vi "Set motor Duty cycle.vi"(8 "error in (no error)":errorcluster, 9 "Tipo de control":T2, 10 "Parametros de control":T1={"Setpoint"=0.0, "PV"=0.0, "Frecuencia PWM"=0.0, "Ciclo de trabajo PWM"=2.5e-06, "V. histeresis (grados)"=0.0, "Ganacias PID"={"proportional gain (Kc)"=1.0, "integral time (Ti, min)"=0.01, "derivative time (Td, min)"=0.0}, "Ref array"=[]} {"Ciclo de trabajo PWM" min=2.5e-06 max=1.0 step=0.1}) -> (0 "error out":errorcluster, 3 "Salida a motores":cluster{"duty cycle":dbl, "frequency":dbl}[](array[cluster]))   [LabVIEW 2018]
uses:
  <vilib>/addons/control/pid/NI_PID_pid.lvlib
  <vilib>/addons/control/pid/pid.llb/PID Percentage to EGU (DBL).vi
  <vilib>/addons/control/pid/_prctrl compat.llb/PID (Compatibility).vi
  <vilib>/addons/control/pid/NI_PID__prctrl compat.lvlib
  typedef/Selector control.ctl
  typedef/Parametros control.ctl
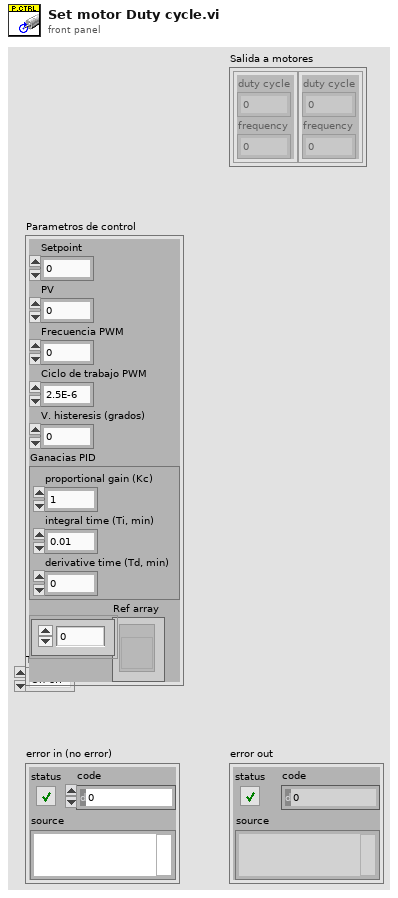
[diagram p1: front panel]
types:
  T1 = typedef "Parametros control.ctl" = cluster{"Setpoint":dbl, "PV":dbl, "Frecuencia PWM":dbl, "Ciclo de trabajo PWM":dbl, "V. histeresis (grados)":dbl, "Ganacias PID":cluster{"proportional gain (Kc)":dbl, "integral time (Ti, min)":dbl, "derivative time (Td, min)":dbl}, "Ref array":refnum<vi>[]}
  T2 = typedef "Selector control.ctl" = enum16{"On-off", "On-off hist.", "PID"}
  T3 = cluster{"sp low":dbl, "sp high":dbl, "out low":dbl, "out high":dbl, "hold (F)":bool, "auto (T)":bool, "pro. band (F)":bool, "reverse acting (T)":bool, "beta":dbl, "linearity":dbl, "dt (s)":dbl}
  T4 = cluster{"proportional gain (Kc)":dbl, "integral time (Ti, min)":dbl, "derivative time (Td, min)":dbl}
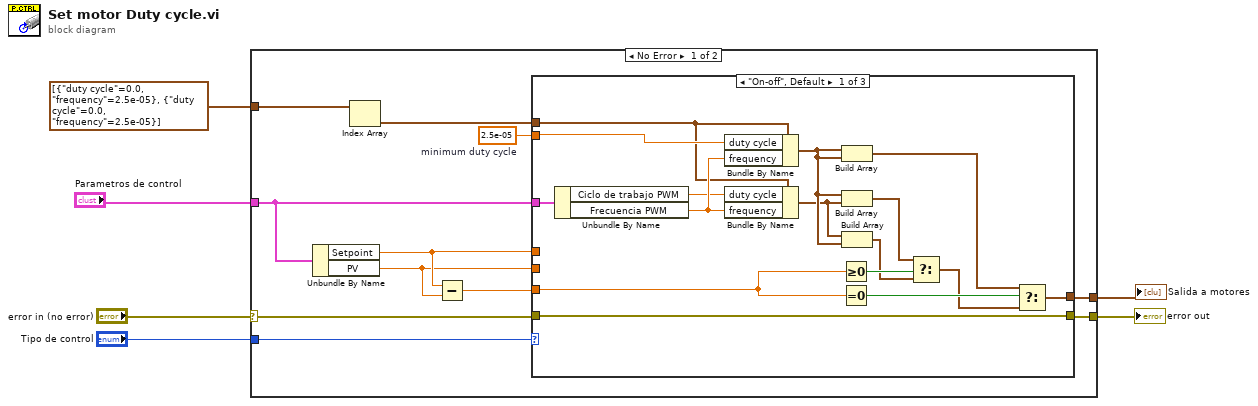
[diagram p0: block diagram]
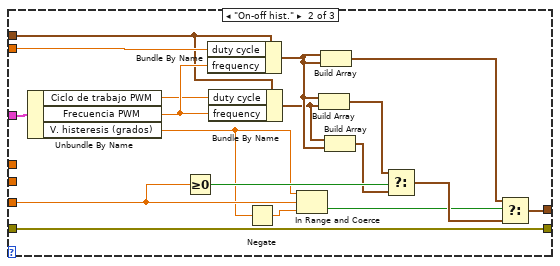
[diagram p2: hidden frame]
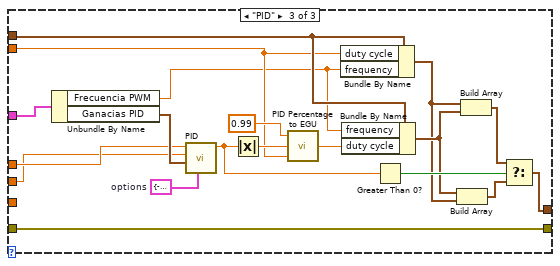
[diagram p3: hidden frame]
diagram:
  n1 = case shown="No Error" "error in (no error)" {
    selector: "error in (no error)" -> [w16 w72]
    tunnel: [w15 w72] -> w5
    tunnel: cluster{"duty cycle":dbl, "frequency":dbl}[] [{"duty cycle"=0.0, "frequency"=2.5e-05}, {"duty cycle"=0.0, "frequency"=2.5e-05}] ("data") -> [w10 w71]
    tunnel: [w17 w71] -> w3
    tunnel: "Parametros de control" -> [w13 _]
    tunnel: "Tipo de control" -> [w14 _]
    frame No Error {
      w11 = 2.5e-05  # minimum duty cycle
      n2 = Unbundle By Name(w13) -> ("Setpoint"=w9:dbl, "PV"=w8:dbl)
      n3 = Index Array(array=w10) -> (element=w7:cluster{"duty cycle":dbl, "frequency":dbl})  [unwired: 1 in]
      n4 = Subtract(x=w9, y=w8) -> (x-y=w12:dbl)
      n5 = case shown="\"On-off\", Default" w14 {
        tunnel: w12 -> [w31 w38 _]
        tunnel: [w22 w42 w63] -> w17
        tunnel: w13 -> [w21 w41 w70]
        tunnel: w16 -> [w20 w40 w68]
        tunnel: [w20 w40 w68] -> w15
        tunnel: w11 -> [w19 w35 w58]
        tunnel: w9 -> [_ _ w60]
        tunnel: w8 -> [_ _ w59]
        tunnel: w7 -> [w18 w34 w66]
        frame "On-off", Default {
          n6 = Unbundle By Name(w21) -> ("Ciclo de trabajo PWM"=w29:dbl, "Frecuencia PWM"=w30:dbl)
          n7 = Bundle By Name(cluster=w18, "duty cycle"=w19, "frequency"=w30) -> (w26:cluster{"duty cycle":dbl, "frequency":dbl})
          n8 = Bundle By Name(cluster=w18, "duty cycle"=w29, "frequency"=w30) -> (w25:cluster{"duty cycle":dbl, "frequency":dbl})
          n9 = Greater Or Equal To 0?(x=w31) -> (x >= 0?=w32:bool)
          n10 = Equal To 0?(x=w31) -> (x = 0?=w33:bool)
          n11 = Build Array(w26, w26) -> (w28:cluster{"duty cycle":dbl, "frequency":dbl}[])
          n12 = Build Array(w26, w25) -> (w27:cluster{"duty cycle":dbl, "frequency":dbl}[])
          n13 = Build Array(w25, w26) -> (w24:cluster{"duty cycle":dbl, "frequency":dbl}[])
          n14 = Select(t=w27, s=w32, f=w24) -> (s? t:f=w23:cluster{"duty cycle":dbl, "frequency":dbl}[])
          n15 = Select(t=w28, s=w33, f=w23) -> (s? t:f=w22:cluster{"duty cycle":dbl, "frequency":dbl}[])
        }
        frame "On-off hist." {
          n16 = Unbundle By Name(w41) -> ("Ciclo de trabajo PWM"=w49:dbl, "Frecuencia PWM"=w50:dbl, "V. histeresis (grados)"=w36:dbl)
          n17 = Greater Or Equal To 0?(x=w38) -> (x >= 0?=w51:bool)
          n18 = Bundle By Name(cluster=w34, "duty cycle"=w35, "frequency"=w50) -> (w46:cluster{"duty cycle":dbl, "frequency":dbl})
          n19 = Bundle By Name(cluster=w34, "duty cycle"=w49, "frequency"=w50) -> (w45:cluster{"duty cycle":dbl, "frequency":dbl})
          n20 = Negate(x=w36) -> (-x=w37:dbl)
          n21 = In Range and Coerce(upper limit=w36, x=w38, lower limit=w37) -> (In Range?=w39:bool)  [unwired: 1 out]
          n22 = Build Array(w46, w45) -> (w47:cluster{"duty cycle":dbl, "frequency":dbl}[])
          n23 = Build Array(w46, w46) -> (w48:cluster{"duty cycle":dbl, "frequency":dbl}[])
          n24 = Build Array(w45, w46) -> (w44:cluster{"duty cycle":dbl, "frequency":dbl}[])
          n25 = Select(t=w47, s=w51, f=w44) -> (s? t:f=w43:cluster{"duty cycle":dbl, "frequency":dbl}[])
          n26 = Select(t=w48, s=w39, f=w43) -> (s? t:f=w42:cluster{"duty cycle":dbl, "frequency":dbl}[])
        }
        frame "PID" {
          w54 = T3 {"sp low"=-180.0, "sp high"=180.0, "out low"=-170.0, "out high"=170.0, "hold (F)"=FALSE, "auto (T)"=TRUE, "pro. band (F)"=FALSE, "reverse acting (T)"=TRUE, "beta"=1.0, "linearity"=1.0, "dt (s)"=-1.0}  # options
          n27 = Unbundle By Name(w70) -> ("Frecuencia PWM"=w53:dbl, "Ganacias PID"=w69:T4)
          n28 = call-poly <vilib>:"PID.vi"("options"=w54, "PID parameters"=w69, "process variable"=w59, "setpoint"=w60) -> ("output"=w62:dbl)  [unwired: 7 in]
          n29 = Absolute Value(x=w62) -> (abs(x)=w61:dbl)
          n30 = call-poly <vilib>:"PID Percentage to EGU.vi"("minimum (EGU)"=w58, "% span"=w61, "maximum (EGU)"=0.99) -> ("output (EGU)"=w52:dbl)  [unwired: 1 in]
          n31 = Bundle By Name(cluster=w66, "duty cycle"=w58, "frequency"=w53) -> (w55:cluster{"duty cycle":dbl, "frequency":dbl})
          n32 = Bundle By Name(cluster=w66, "frequency"=w53, "duty cycle"=w52) -> (w64:cluster{"duty cycle":dbl, "frequency":dbl})
          n33 = Greater Than 0?(x=w62) -> (x > 0?=w65:bool)
          n34 = Build Array(w64, w55) -> (w56:cluster{"duty cycle":dbl, "frequency":dbl}[])
          n35 = Build Array(w55, w64) -> (w57:cluster{"duty cycle":dbl, "frequency":dbl}[])
          n36 = Select(t=w57, s=w65, f=w56) -> (s? t:f=w63:cluster{"duty cycle":dbl, "frequency":dbl}[])
        }
      }
    }
    frame Error {
    }
  }
  "error out" <- w5
  "Salida a motores" <- w3
